vi "PH_DeformableMirror.set GUI Elements.vi"(0 "VI in":refnum<vi>, 5 "error in (no error)":errorcluster) -> (14 "VI out":refnum<vi>, 19 "error out":errorcluster)   [LabVIEW 2014, in "PH_DeformableMirror.lvlib"]
uses:
  PH_DeformableMirror.lvlib
  instr.lib/dmdriver/DMirrorBase/DMirrorBase.lvclass/DMirrorBase.ctl
  instr.lib/dmdriver/DMirrorBase/IsInitialized.vi
  instr.lib/dmdriver/DMirrorBase/Read #of channels.vi
  instr.lib/dmdriver/DMirrorBase/Get valid value range.vi
  instr.lib/dmdriver/DMirrorBase/DMirrorBase.lvclass
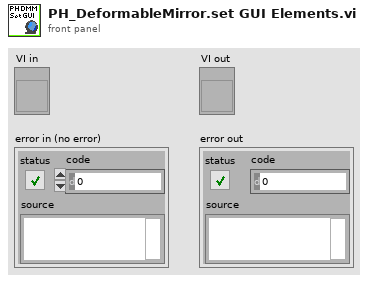
[diagram p1: front panel]
types:
  T1 = typedef "PH_DeformableMirror.lvlib/PH_DeformableMirror.i attribute.ctl" = cluster{"DMirror.lvlib:DMirrorBase.lvclass":refnum<class "DMirrorBase.lvclass">, "Device error":errorcluster, "GUI Refs":cluster{"Delete":refnum<vi>, "Device Error":refnum<vi>, "HV on":refnum<vi>, "Channel":refnum<vi>, "Voltage":refnum<vi>, "Channel Voltages":refnum<vi>}}
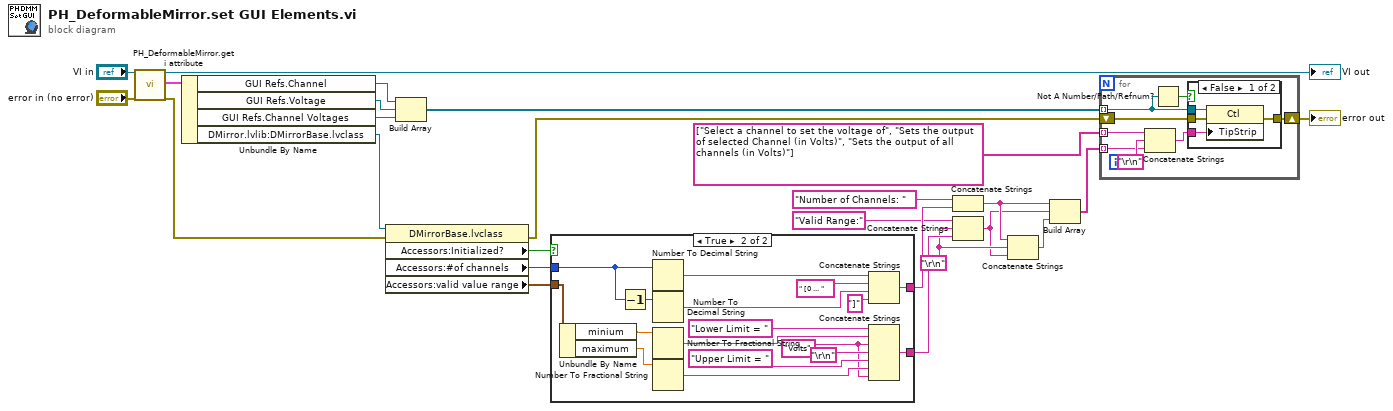
[diagram p0: block diagram]
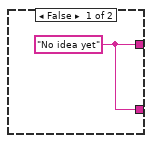
[diagram p2: hidden frame]
diagram:
  w4 = "\r\n"
  n1 = call "PH_DeformableMirror.get i attribute.vi"("i ref in"="VI in", "error in (no error)"="error in (no error)") -> ("i ref out"=→"VI out":refnum<vi>, "i attribute"=w23:T1, "error out"=w22:errorcluster)  [unwired: 15 in]
  n2 = Unbundle By Name(w23) -> ("GUI Refs.Channel"=w16:refnum<vi>, "GUI Refs.Voltage"=w17:refnum<vi>, "GUI Refs.Channel Voltages"=w18:refnum<vi>, "DMirror.lvlib:DMirrorBase.lvclass"=w14:refnum<class "DMirrorBase.lvclass">)
  n3 = property class="DMirrorBase.lvclass"(reference=w14, error in=w22) -> (error out=w20:errorcluster, "Accessors:Initialized?"=w7:bool, "Accessors:#of channels"=w12:u32, "Accessors:valid value range"=w13:cluster{"minium":dbl, "maximum":dbl})  [unwired: 1 out]
  n4 = Build Array(w16, w17, w18) -> (w15:refnum<vi>[])
  n5 = case shown="True" w7 {
    tunnel: w13 -> [_ w43]
    tunnel: w12 -> [_ w31]
    tunnel: [w26 w28] -> w10
    tunnel: [w26 w27] -> w8
    frame False {
      w26 = "No idea yet"
    }
    frame True {
      w35 = "Volts" ("string")
      n6 = Unbundle By Name(w43) -> ("minium"=w41:dbl, "maximum"=w40:dbl)
      n7 = Decrement(x=w31) -> (x-1=w30:u32)
      n8 = Number To Decimal String(number=w31) -> (decimal integer string=w34:string)  [unwired: 1 in]
      n9 = Number To Decimal String(number=w30) -> (decimal integer string=w29:string)  [unwired: 1 in]
      n10 = Number To Fractional String(number=w41) -> (F-format string=w39:string)  [unwired: 3 in]
      n11 = Number To Fractional String(number=w40) -> (F-format string=w36:string)  [unwired: 3 in]
      n12 = Concatenate Strings(w34, " [0 ... " ("string"), w29, "]" ("string")) -> (w28:string)
      n13 = Concatenate Strings("Lower Limit = ", w39, w35, "\r\n", "Upper Limit = " ("string"), w36, w35) -> (w27:string)
    }
  }
  n14 = Concatenate Strings("Number of Channels: " ("string"), w10) -> (w5:string)
  n15 = Concatenate Strings("Valid Range:" ("string"), w4, w8) -> (w3:string)
  n16 = Concatenate Strings(w5, w4, w3) -> (w2:string)
  n17 = Build Array(w5, w3, w2) -> (w1:string[])
  n18 = for {
    shift-right: [w50] -> w21
    shift-left: w20 -> [w51]
    tunnel: w15 -> [w48] mode=indexing
    tunnel: string[] ["Select a channel to set the voltage of", "Sets the output of selected Channel (in Volts)", "Sets the output of all channels (in Volts)"] -> [w46] mode=indexing
    tunnel: w1 -> [w44] mode=indexing
    n19 = Concatenate Strings(w46, "\r\n", w44) -> (w47:string)
    n20 = Not A Number/Path/Refnum?(number/path/refnum=w48) -> (NaN/Path/Refnum?=w49:bool)
    n21 = case shown="False" w49 {
      tunnel: w51 -> [w55 w56]
      tunnel: [w54 w56] -> w50
      tunnel: w48 -> [w53 _]
      tunnel: w47 -> [w52 _]
      frame False {
        n22 = property class="Ctl"(reference=w53, error in=w55, "TipStrip"=w52) -> (error out=w54:errorcluster)  [unwired: 1 out]
      }
      frame True {
      }
    }
  }
  "error out" <- w21
